vi "Get Version Independent.vi"(8 "error in (no error)":errorcluster, 11 "NI_AB_API_Targetfile in":refnum<class "NI_AB_API_Targetfile.lvclass">) -> (0 "error out":errorcluster, 2 "versionIndependent":bool, 3 "NI_AB_API_Targetfile out":refnum<class "NI_AB_API_Targetfile.lvclass">)   [LabVIEW 2020, in "NI_AB_API_Targetfile.lvclass"]
uses:
  <vilib>/AppBuilder/AB_API/Targetfile/NI_AB_API_Targetfile.lvclass
  e:/builds/penguin/labview/branches/2020/dev/dist/vi.lib/AppBuilder/AB_API/Build/NI_AB_API_Build.lvclass
  <vilib>/AppBuilder/AB_Classes/TargetFile/AB_Targetfile.lvclass
  <vilib>/AppBuilder/AB_API/Build/NI_AB_API_Build.lvclass
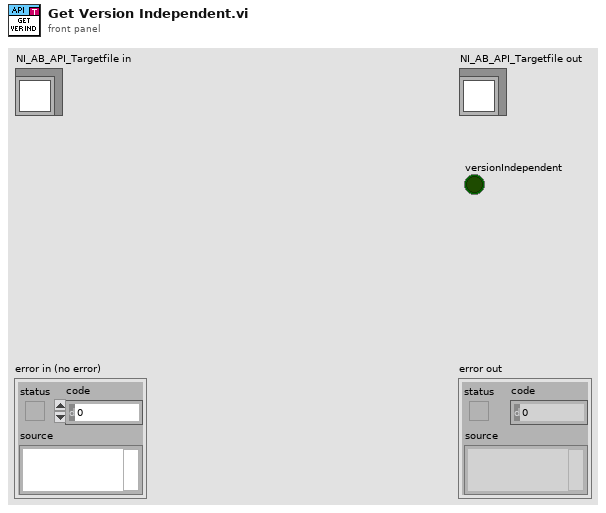
[diagram p1: front panel]
types:
  T1 = typedef "AB_Targetfile.ctl" = cluster{"targetfileName":string, "targetfileGUID":string, "enableDebugging":bool, "versionInfo":cluster{"productName":string, "legalCopyright":string, "companyName":string, "internalName":string, "fileDescription":string}, "eng_consolidatedTypeInfo":string, "fastFileFormat":bool, "eng_LEIFBuildData":u32, "versionIndependent":bool}
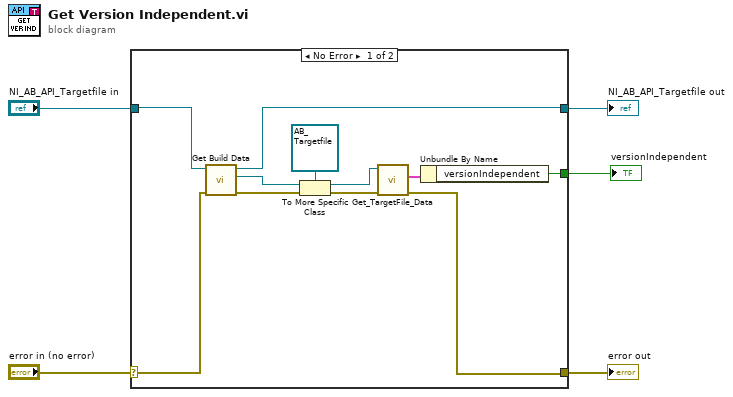
[diagram p0: block diagram]
diagram:
  n1 = case shown="No Error" "error in (no error)" {
    selector: "error in (no error)" -> [w10 w18]
    tunnel: [w8 w18] -> w4
    tunnel: [w9 w17] -> w2
    tunnel: "NI_AB_API_Targetfile in" -> [w11 w17]
    tunnel: [w6 _] -> w1
    frame No Error {
      n2 = call <vilib>:"Get Build Data.vi"("error in (no error)"=w10, "NI_AB_API_Build in"=w11) -> ("error out"=w13:errorcluster, "AB_Build.lvclass"=w15:refnum<class "AB_Build.lvclass">, "NI_AB_API_Build out"=w9:refnum<class "NI_AB_API_Targetfile.lvclass">)  [unwired: 7 in]
      n3 = To More Specific Class(target class=refnum<class "AB_Targetfile.lvclass"> refnum ("AB_Targetfile in"), reference=w15, error in=w13) -> (specific class reference=w14:refnum<class "AB_Targetfile.lvclass">, error out=w12:errorcluster)
      n4 = call <vilib>:"Get_TargetFile_Data.vi"("error in (no error)"=w12, "AB_Targetfile in"=w14) -> ("error out"=w8:errorcluster, "data"=w7:T1)  [unwired: 7 in, 1 out]
      n5 = Unbundle By Name(w7) -> ("versionIndependent"=w6:bool)
    }
    frame Error {
    }
  }
  "error out" <- w4
  "NI_AB_API_Targetfile out" <- w2
  "versionIndependent" <- w1
